vi "test_read-nmea-data2.vi"() -> ()   [LabVIEW 2019] (continued)
,1,04,11,50,132,25,14,87,127,24,28,,,21,33,60,219,29,1*46\n\t\n15:12:35.67\tF9P\t$GBGSV,1,1,03,11,50,132,,14,87,127,33,33,60,219,,3*40\n\t\n15:12:35.69\tF9P\t$GNGLL,3723.54317,N,12656.94702,E,061237.00,A,A*79\n\t\n15:12:35.71\tF9P\t\t\n15:12:35.73\tF9P\t\t\n15:12:35.75\tF9P\t\t\n15:12:35.77\tF9P\t\t\n15:12:35.79\tF9P\t\t\n15:12:35.81\tF9P\t\t\n15:12:35.83\tF9P\t\t\n15:12:35.85\tF9P\t\t\n15:12:35.87\tF9P\t\t\n15:12:35.89\tF9P\t\t\n15:12:35.91\tF9P\t\t\n15:12:35.93\tF9P\t\t\n15:12:35.95\tF9P\t\t\n15:12:35.97\tF9P\t\t\n15:12:35.99\tF9P\t\t\n15:12:36.01\tF9P\t\t\n15:12:36.03\tF9P\t\t\n15:12:36.05\tF9P\t\t\n15:12:36.07\tF9P\t\t\n15:12:36.09\tF9P\t\t\n15:12:36.11\tF9P\t\t\n15:12:36.13\tF9P\t\t\n15:12:36.15\tF9P\t\t\n15:12:36.17\tF9P\t\t\n15:12:36.19\tF9P\t\t\n15:12:36.21\tF9P\t\t\n15:12:36.23\tF9P\t$GNRMC,061238.00,A,3723.54347,N,12656.94820,E,2.767,70.74,250720,,,A,V*33\n\t\n15:12:36.25\tF9P\t$GNVTG,70.74,T,,M,2.767,N,5.124,K,A*11\n\t\n15:12:36.27\tF9P\t$GNGGA,061238.00,3723.54347,N,12656.94820,E,1,12,0.86,47.3,M,18.5,M,,*78\n\t\n15:12:36.29\tF9P\t$GNGSA,A,3,12,06,19,05,17,09,04,02,,,,,1.43,0.86,1.14,1*0C\n\t\n15:12:36.31\tF9P\t$GNGSA,A,3,85,70,71,84,,,,,,,,,1.43,0.86,1.14,2*0E\n\t\n15:12:36.33\tF9P\t$GNGSA,A,3,36,19,11,04,09,12,,,,,,,1.43,0.86,1.14,3*0C\n\t\n15:12:36.35\tF9P\t$GNGSA,A,3,14,11,33,,,,,,,,,,1.43,0.86,1.14,4*0D\n\t\n15:12:36.37\tF9P\t$GPGSV,3,1,09,02,55,319,20,04,18,043,24,05,37,247,38,06,64,049,28,1*60\n\t\n15:12:36.39\tF9P\t$GPGSV,3,2,09,09,45,074,32,12,23,276,30,17,33,154,35,19,52,157,30,1*6B\n\t\n15:12:36.41\tF9P\t$GPGSV,3,3,09,25,12,306,,1*5C\n\t\n15:12:36.43\tF9P\t$GPGSV,3,1,09,02,55,319,,04,18,043,18,05,37,247,21,06,64,049,28,6*62\n\t\n15:12:36.45\tF9P\t$GPGSV,3,2,09,09,45,074,29,12,23,276,16,17,33,154,27,19,52,157,,6*62\n\t\n15:12:36.47\tF9P\t$GPGSV,3,3,09,25,12,306,,6*5B\n\t\n15:12:36.49\tF9P\t$GLGSV,2,1,08,69,12,031,,70,71,039,33,71,52,205,38,72,04,209,23,1*70\n\t\n15:12:36.51\tF9P\t$GLGSV,2,2,08,77,01,326,,84,20,122,10,85,70,067,41,86,37,330,,1*7C\n\t\n15:12:36.53\tF9P\t$GLGSV,2,1,08,69,12,031,,70,71,039,,71,52,205,24,72,04,209,,3*7E\n\t\n15:12:36.55\tF9P\t$GLGSV,2,2,08,77,01,326,,84,20,122,15,85,70,067,21,86,37,330,,3*7D\n\t\n15:12:36.57\tF9P\t$GAGSV,2,1,08,02,08,297,07,04,66,116,32,09,32,193,39,11,72,359,27,7*7C\n\t\n15:12:36.59\tF9P\t$GAGSV,2,2,08,12,40,103,24,19,26,045,17,25,09,249,,36,26,308,21,7*7B\n\t\n15:12:36.61\tF9P\t$GAGSV,2,1,08,02,08,297,,04,66,116,,09,32,193,,11,72,359,,2*70\n\t\n15:12:36.63\tF9P\t$GAGSV,2,2,08,12,40,103,,19,26,045,,25,09,249,,36,26,308,,2*7D\n\t\n15:12:36.65\tF9P\t$GBGSV,1,1,04,11,50,132,26,14,87,127,26,28,,,20,33,60,219,36,1*48\n\t\n15:12:36.67\tF9P\t$GBGSV,1,1,03,11,50,132,,14,87,127,28,33,60,219,,3*4A\n\t\n15:12:36.69\tF9P\t$GNGLL,3723.54347,N,12656.94820,E,061238.00,A,A*7C\n\t\n15:12:36.71\tF9P\t\t\n15:12:36.73\tF9P\t\t\n15:12:36.75\tF9P\t\t\n15:12:36.78\tF9P\t\t\n15:12:36.80\tF9P\t\t\n15:12:36.82\tF9P\t\t\n15:12:36.84\tF9P\t\t\n15:12:36.86\tF9P\t\t\n15:12:36.88\tF9P\t\t\n15:12:36.90\tF9P\t\t\n15:12:36.92\tF9P\t\t\n15:12:36.94\tF9P\t\t\n15:12:36.96\tF9P\t\t\n15:12:36.98\tF9P\t\t\n15:12:37.00\tF9P\t\t\n15:12:37.02\tF9P\t\t\n15:12:37.04\tF9P\t\t\n15:12:37.06\tF9P\t\t\n15:12:37.08\tF9P\t\t\n15:12:37.10\tF9P\t\t\n15:12:37.12\tF9P\t\t\n15:12:37.14\tF9P\t\t\n15:12:37.16\tF9P\t\t\n15:12:37.18\tF9P\t\t\n15:12:37.20\tF9P\t\t\n15:12:37.22\tF9P\t\t\n15:12:37.24\tF9P\t$GNRMC,061239.00,A,3723.54405,N,12656.94928,E,3.255,61.63,250720,,,A,V*39\n\t\n15:12:37.26\tF9P\t$GNVTG,61.63,T,,M,3.255,N,6.028,K,A*1C\n\t\n15:12:37.28\tF9P\t$GNGGA,061239.00,3723.54405,N,12656.94928,E,1,12,0.86,46.9,M,18.5,M,,*7A\n\t\n15:12:37.30\tF9P\t$GNGSA,A,3,12,06,19,05,17,09,04,02,,,,,1.43,0.86,1.14,1*0C\n\t\n15:12:37.32\tF9P\t$GNGSA,A,3,85,70,71,84,,,,,,,,,1.43,0.86,1.14,2*0E\n\t\n15:12:37.34\tF9P\t$GNGSA,A,3,36,19,11,04,09,12,,,,,,,1.43,0.86,1.14,3*0C\n\t\n15:12:37.36\tF9P\t$GNGSA,A,3,14,11,33,,,,,,,,,,1.43,0.86,1.14,4*0D\n\t\n15:12:37.38\tF9P\t$GPGSV,3,1,09,02,55,319,23,04,18,043,24,05,37,247,35,06,64,049,31,1*66\n\t\n15:12:37.40\tF9P\t$GPGSV,3,2,09,09,45,074,30,12,23,276,29,17,33,154,29,19,52,157,34,1*68\n\t\n15:12:37.42\tF9P\t$GPGSV,3,3,09,25,12,306,25,1*5B\n\t\n15:12:37.44\tF9P\t$GPGSV,3,1,09,02,55,319,,04,18,043,19,05,37,247,20,06,64,049,28,6*62\n\t\n15:12:37.46\tF9P\t$GPGSV,3,2,09,09,45,074,32,12,23,276,16,17,33,154,26,19,52,157,,6*69\n\t\n15:12:37.48\tF9P\t$GPGSV,3,3,09,25,12,306,,6*5B\n\t\n15:12:37.50\tF9P\t$GLGSV,2,1,08,69,12,031,,70,71,039,33,71,52,205,43,72,04,209,22,1*7D\n\t\n15:12:37.52\tF9P\t$GLGSV,2,2,08,77,01,326,,84,20,122,14,85,70,067,36,86,37,330,,1*78\n\t\n15:12:37.54\tF9P\t$GLGSV,2,1,08,69,12,031,,70,71,039,,71,52,205,24,72,04,209,,3*7E\n\t\n15:12:37.56\tF9P\t$GLGSV,2,2,08,77,01,326,,84,20,122,16,85,70,067,29,86,37,330,,3*76\n\t\n15:12:37.58\tF9P\t$GAGSV,2,1,08,02,08,297,13,04,66,116,27,09,32,193,33,11,72,359,32,7*73\n\t\n15:12:37.60\tF9P\t$GAGSV,2,2,08,12,40,103,35,19,26,045,17,25,09,249,,36,26,308,24,7*7E\n\t\n15:12:37.62\tF9P\t$GAGSV,2,1,08,02,08,297,,04,66,116,,09,32,193,,11,72,359,,2*70\n\t\n15:12:37.64\tF9P\t$GAGSV,2,2,08,12,40,103,,19,26,045,,25,09,249,,36,26,308,,2*7D\n\t\n15:12:37.66\tF9P\t$GBGSV,1,1,04,11,50,132,27,14,87,127,32,28,,,21,33,60,219,37,1*4C\n\t\n15:12:37.68\tF9P\t$GBGSV,1,1,03,11,50,132,,14,87,127,28,33,60,219,,3*4A\n\t\n15:12:37.70\tF9P\t$GNGLL,3723.54405,N,12656.94928,E,061239.00,A,A*75\n\t\n15:12:37.72\tF9P\t\t\n15:12:37.74\tF9P\t\t\n15:12:37.76\tF9P\t\t\n15:12:37.78\tF9P\t\t\n15:12:37.80\tF9P\t\t\n15:12:37.82\tF9P\t\t\n15:12:37.84\tF9P\t\t\n15:12:37.86\tF9P\t\t\n15:12:37.88\tF9P\t\t\n15:12:37.90\tF9P\t\t\n15:12:37.92\tF9P\t\t\n15:12:37.94\tF9P\t\t\n15:12:37.96\tF9P\t\t\n15:12:37.98\tF9P\t\t\n15:12:38.00\tF9P\t\t\n15:12:38.02\tF9P\t\t\n15:12:38.04\tF9P\t\t\n15:12:38.06\tF9P\t\t\n15:12:38.08\tF9P\t\t\n15:12:38.10\tF9P\t\t\n15:12:38.12\tF9P\t\t\n15:12:38.14\tF9P\t\t\n15:12:38.16\tF9P\t\t\n15:12:38.18\tF9P\t\t\n15:12:38.20\tF9P\t\t\n15:12:38.22\tF9P\t\t\n15:12:38.24\tF9P\t$GNRMC,061240.00,A,3723.54439,N,12656.95015,E,2.349,62.25,250720,,,A,V*32\n\t\n15:12:38.26\tF9P\t$GNVTG,62.25,T,,M,2.349,N,4.351,K,A*1F\n\t\n15:12:38.28\tF9P\t$GNGGA,061240.00,3723.54439,N,12656.95015,E,1,12,0.90,47.7,M,18.5,M,,*75\n\t\n15:12:38.30\tF9P\t$GNGSA,A,3,12,06,19,05,17,09,04,02,,,,,1.51,0.90,1.21,1*0E\n\t\n15:12:38.32\tF9P\t$GNGSA,A,3,85,70,71,84,,,,,,,,,1.51,0.90,1.21,2*0C\n\t\n15:12:38.34\tF9P\t$GNGSA,A,3,36,19,11,04,09,12,,,,,,,1.51,0.90,1.21,3*0E\n\t\n15:12:38.36\tF9P\t$GNGSA,A,3,14,11,33,,,,,,,,,,1.51,0.90,1.21,4*0F\n\t\n15:12:38.38\tF9P\t$GPGSV,3,1,09,02,55,319,25,04,18,043,23,05,37,247,29,06,64,049,32,1*69\n\t\n15:12:38.40\tF9P\t$GPGSV,3,2,09,09,45,074,29,12,23,276,21,17,33,154,36,19,52,157,33,1*61\n\t\n15:12:38.42\tF9P\t$GPGSV,3,3,09,25,12,306,22,1*5C\n\t\n15:12:38.44\tF9P\t$GPGSV,3,1,09,02,55,319,,04,18,043,17,05,37,247,21,06,64,049,28,6*6D\n\t\n15:12:38.46\tF9P\t$GPGSV,3,2,09,09,45,074,27,12,23,276,14,17,33,154,25,19,52,157,,6*6C\n\t\n15:12:38.48\tF9P\t$GPGSV,3,3,09,25,12,306,,6*5B\n\t\n15:12:38.50\tF9P\t$GLGSV,2,1,08,69,12,031,,70,71,039,33,71,52,205,45,72,04,209,20,1*79\n\t\n15:12:38.52\tF9P\t$GLGSV,2,2,08,77,01,326,,84,20,122,10,85,70,067,32,86,37,330,,1*78\n\t\n15:12:38.54\tF9P\t$GLGSV,2,1,08,69,12,031,,70,71,039,,71,52,205,24,72,04,209,,3*7E\n\t\n15:12:38.56\tF9P\t$GLGSV,2,2,08,77,01,326,,84,20,122,17,85,70,067,24,86,37,330,,3*7A\n\t\n15:12:38.58\tF9P\t$GAGSV,2,1,08,02,08,297,12,04,66,116,27,09,32,193,30,11,72,359,31,7*72\n\t\n15:12:38.60\tF9P\t$GAGSV,2,2,08,12,40,103,31,19,26,045,17,25,09,249,,36,26,308,23,7*7D\n\t\n15:12:38.62\tF9P\t$GAGSV,2,1,08,02,08,297,,04,66,116,,09,32,193,,11,72,359,,2*70\n\t\n15:12:38.64\tF9P\t$GAGSV,2,2,08,12,40,103,,19,26,045,,25,09,249,,36,26,308,,2*7D\n\t\n15:12:38.66\tF9P\t$GBGSV,1,1,04,11,50,132,28,14,87,127,28,28,,,23,33,60,219,31,1*4C\n\t\n15:12:38.68\tF9P\t$GBGSV,1,1,03,11,50,132,,14,87,127,26,33,60,219,,3*44\n\t\n15:12:38.70\tF9P\t$GNGLL,3723.54439,N,12656.95015,E,061240.00,A,A*72\n\t\n15:12:38.72\tF9P\t\t\n15:12:38.74\tF9P\t\t\n15:12:38.76\tF9P\t\t\n15:12:38.78\tF9P\t\t\n15:12:38.80\tF9P\t\t\n15:12:38.82\tF9P\t\t\n15:12:38.84\tF9P\t\t\n15:12:38.86\tF9P\t\t\n15:12:38.88\tF9P\t\t\n15:12:38.90\tF9P\t\t\n15:12:38.92\tF9P\t\t\n15:12:38.94\tF9P\t\t\n15:12:38.96\tF9P\t\t\n15:12:38.98\tF9P\t\t\n15:12:39.00\tF9P\t\t\n15:12:39.02\tF9P\t\t\n15:12:39.04\tF9P\t\t\n15:12:39.06\tF9P\t\t\n15:12:39.08\tF9P\t\t\n15:12:39.10\tF9P\t\t\n15:12:39.12\tF9P\t\t\n15:12:39.14\tF9P\t\t\n15:12:39.16\tF9P\t\t\n15:12:39.18\tF9P\t\t\n15:12:39.20\tF9P\t\t\n15:12:39.22\tF9P\t\t\n15:12:39.24\tF9P\t$GNRMC,061241.00,A,3723.54500,N,12656.95069,E,3.058,25.00,250720,,,A,V*35\n\t\n15:12:39.26\tF9P\t$GNVTG,25.00,T,,M,3.058,N,5.663,K,A*1C\n\t\n15:12:39.28\tF9P\t$GNGGA,061241.00,3723.54500,N,12656.95069,E,1,12,0.82,49.2,M,18.5,M,,*7C\n\t\n15:12:39.30\tF9P\t$GNGSA,A,3,12,06,19,05,17,09,04,02,,,,,1.45,0.82,1.20,1*09\n\t\n15:12:39.32\tF9P\t$GNGSA,A,3,85,70,71,84,,,,,,,,,1.45,0.82,1.20,2*0B\n\t\n15:12:39.34\tF9P\t$GNGSA,A,3,36,19,11,04,09,12,,,,,,,1.45,0.82,1.20,3*09\n\t\n15:12:39.36\tF9P\t$GNGSA,A,3,14,11,33,,,,,,,,,,1.45,0.82,1.20,4*08\n\t\n15:12:39.38\tF9P\t$GPGSV,3,1,09,02,55,319,32,04,18,043,23,05,37,247,33,06,64,049,33,1*65\n\t\n15:12:39.40\tF9P\t$GPGSV,3,2,09,09,45,074,30,12,23,276,21,17,33,154,33,19,52,157,26,1*68\n\t\n15:12:39.42\tF9P\t$GPGSV,3,3,09,25,12,306,21,1*5F\n\t\n15:12:39.44\tF9P\t$GPGSV,3,1,09,02,55,319,,04,18,043,16,05,37,247,21,06,64,049,29,6*6D\n\t\n15:12:39.46\tF9P\t$GPGSV,3,2,09,09,45,074,32,12,23,276,12,17,33,154,25,19,52,157,,6*6E\n\t\n15:12:39.48\tF9P\t$GPGSV,3,3,09,25,12,306,,6*5B\n\t\n15:12:39.50\tF9P\t$GLGSV,2,1,08,69,12,031,,70,71,039,33,71,52,205,38,72,04,209,23,1*70\n\t\n15:12:39.52\tF9P\t$GLGSV,2,2,08,77,01,326,,84,20,122,08,85,70,067,38,86,37,330,,1*7B\n\t\n15:12:39.54\tF9P\t$GLGSV,2,1,08,69,12,031,,70,71,039,,71,52,205,22,72,04,209,,3*78\n\t\n15:12:39.56\tF9P\t$GLGSV,2,2,08,77,01,326,,84,20,122,17,85,70,067,23,86,37,330,,3*7D\n\t\n15:12:39.58\tF9P\t$GAGSV,2,1,08,02,08,297,11,04,66,116,26,09,32,193,31,11,72,359,32,7*72\n\t\n15:12:39.60\tF9P\t$GAGSV,2,2,08,12,40,103,31,19,26,045,16,25,09,249,,36,26,308,22,7*7D\n\t\n15:12:39.62\tF9P\t$GAGSV,2,1,08,02,08,297,,04,66,116,,09,32,193,,11,72,359,,2*70\n\t\n15:12:39.64\tF9P\t$GAGSV,2,2,08,12,40,103,,19,26,045,,25,09,249,,36,26,308,,2*7D\n\t\n15:12:39.66\tF9P\t$GBGSV,1,1,04,11,50,132,26,14,87,127,28,28,,,29,33,60,219,33,1*4A\n\t\n15:12:39.68\tF9P\t$GBGSV,1,1,03,11,50,132,,14,87,127,30,33,60,219,,3*43\n\t\n15:12:39.70\tF9P\t$GNGLL,3723.54500,N,12656.95069,E,061241.00,A,A*73\n\t\n15:12:39.72\tF9P\t\t\n15:12:39.74\tF9P\t\t\n15:12:39.76\tF9P\t\t\n15:12:39.78\tF9P\t\t\n15:12:39.80\tF9P\t\t\n15:12:39.82\tF9P\t\t\n15:12:39.84\tF9P\t\t\n15:12:39.86\tF9P\t\t\n15:12:39.88\tF9P\t\t\n15:12:39.90\tF9P\t\t\n15:12:39.92\tF9P\t\t\n15:12:39.94\tF9P\t\t\n15:12:39.96\tF9P\t\t\n15:12:39.98\tF9P\t\t\n15:12:40.00\tF9P\t\t\n15:12:40.02\tF9P\t\t\n15:12:40.04\tF9P\t\t\n15:12:40.06\tF9P\t\t\n15:12:40.08\tF9P\t\t\n15:12:40.10\tF9P\t\t\n15:12:40.12\tF9P\t\t\n15:12:40.14\tF9P\t\t\n15:12:40.16\tF9P\t\t\n15:12:40.18\tF9P\t\t\n15:12:40.20\tF9P\t\t\n15:12:40.22\tF9P\t\t\n15:12:40.24\tF9P\t$GNRMC,061242.00,A,3723.54545,N,12656.95138,E,2.338,43.76,250720,,,A,V*37\n\t\n15:12:40.26\tF9P\t$GNVTG,43.76,T,,M,2.338,N,4.331,K,A*1A\n\t\n15:12:40.28\tF9P\t$GNGGA,061242.00,3723.54545,N,12656.95138,E,1,12,0.82,49.2,M,18.5,M,,*7B\n\t\n15:12:40.30\tF9P\t$GNGSA,A,3,12,06,19,05,17,09,04,02,,,,,1.45,0.82,1.20,1*09\n\t\n15:12:40.32\tF9P\t$GNGSA,A,3,85,70,71,84,,,,,,,,,1.45,0.82,1.20,2*0B\n\t\n15:12:40.34\tF9P\t$GNGSA,A,3,36,19,11,04,09,12,,,,,,,1.45,0.82,1.20,3*09\n\t\n15:12:40.36\tF9P\t$GNGSA,A,3,14,11,33,,,,,,,,,,1.45,0.82,1.20,4*08\n\t\n15:12:40.38\tF9P\t$GPGSV,3,1,09,02,55,319,39,04,18,043,29,05,37,247,36,06,64,049,31,1*63\n\t\n15:12:40.40\tF9P\t$GPGSV,3,2,09,09,45,074,33,12,23,276,23,17,33,154,33,19,52,157,35,1*6B\n\t\n15:12:40.42\tF9P\t$GPGSV,3,3,09,25,12,306,20,1*5E\n\t\n15:12:40.44\tF9P\t$GPGSV,3,1,09,02,55,319,,04,18,043,15,05,37,247,22,06,64,049,28,6*6C\n\t\n15:12:40.46\tF9P\t$GPGSV,3,2,09,09,45,074,28,12,23,276,14,17,33,154,25,19,52,157,,6*63\n\t\n15:12:40.48\tF9P\t$GPGSV,3,3,09,25,12,306,,6*5B\n\t\n15:12:40.50\tF9P\t$GLGSV,2,1,08,69,12,031,23,70,71,039,33,71,52,205,43,72,04,209,23,1*7D\n\t\n15:12:40.52\tF9P\t$GLGSV,2,2,08,77,01,326,,84,20,122,11,85,70,067,33,86,37,330,,1*78\n\t\n15:12:40.54\tF9P\t$GLGSV,2,1,08,69,12,031,,70,71,039,,71,52,205,20,72,04,209,,3*7A\n\t\n15:12:40.56\tF9P\t$GLGSV,2,2,08,77,01,326,,84,20,122,18,85,70,067,29,86,37,330,,3*78\n\t\n15:12:40.58\tF9P\t$GAGSV,2,1,08,02,08,297,14,04,66,116,26,09,32,193,35,11,72,359,35,7*74\n\t\n15:12:40.60\tF9P\t$GAGSV,2,2,08,12,40,103,26,19,26,045,15,25,09,249,,36,26,308,20,7*7A\n\t\n15:12:40.62\tF9P\t$GAGSV,2,1,08,02,08,297,,04,66,116,,09,32,193,,11,72,359,,2*70\n\t\n15:12:40.64\tF9P\t$GAGSV,2,2,08,12,40,103,,19,26,045,,25,09,249,,36,26,308,,2*7D\n\t\n15:12:40.66\tF9P\t$GBGSV,1,1,04,11,50,132,26,14,87,127,29,28,,,38,33,60,219,34,1*4C\n\t\n15:12:40.68\tF9P\t$GBGSV,1,1,03,11,50,132,,14,87,127,29,33,60,219,,3*4B\n\t\n15:12:40.70\tF9P\t$GNGLL,3723.54545,N,12656.95138,E,061242.00,A,A*74\n\t\n15:12:40.72\tF9P\t\t\n15:12:40.74\tF9P\t\t\n15:12:40.76\tF9P\t\t\n15:12:40.78\tF9P\t\t\n15:12:40.80\tF9P\t\t\n15:12:40.82\tF9P\t\t\n15:12:40.84\tF9P\t\t\n15:12:40.86\tF9P\t\t\n15:12:40.88\tF9P\t\t\n15:12:40.90\tF9P\t\t\n15:12:40.92\tF9P\t\t\n15:12:40.94\tF9P\t\t\n15:12:40.96\tF9P\t\t\n15:12:40.98\tF9P\t\t\n15:12:41.00\tF9P\t\t\n15:12:41.02\tF9P\t\t\n15:12:41.04\tF9P\t\t\n15:12:41.06\tF9P\t\t\n15:12:41.08\tF9P\t\t\n15:12:41.10\tF9P\t\t\n15:12:41.12\tF9P\t\t\n15:12:41.14\tF9P\t\t\n15:12:41.16\tF9P\t\t\n15:12:41.18\tF9P\t\t\n15:12:41.20\tF9P\t\t\n15:12:41.22\tF9P\t\t\n15:12:41.24\tF9P\t$GNRMC,061243.00,A,3723.54595,N,12656.95226,E,2.215,50.75,250720,,,A,V*38\n\t\n15:12:41.26\tF9P\t$GNVTG,50.75,T,,M,2.215,N,4.102,K,A*17\n\t\n15:12:41.28\tF9P\t$GNGGA,061243.00,3723.54595,N,12656.95226,E,1,12,0.82,48.7,M,18.5,M,,*7F\n\t\n15:12:41.30\tF9P\t$GNGSA,A,3,12,06,19,05,17,09,04,02,,,,,1.45,0.82,1.20,1*09\n\t\n15:12:41.32\tF9P\t$GNGSA,A,3,85,70,71,84,,,,,,,,,1.45,0.82,1.20,2*0B\n\t\n15:12:41.34\tF9P\t$GNGSA,A,3,36,19,11,04,09,12,,,,,,,1.45,0.82,1.20,3*09\n\t\n15:12:41.36\tF9P\t$GNGSA,A,3,14,11,33,,,,,,,,,,1.45,0.82,1.20,4*08\n\t\n15:12:41.38\tF9P\t$GPGSV,3,1,09,02,55,319,43,04,18,043,27,05,37,247,37,06,64,049,25,1*64\n\t\n15:12:41.40\tF9P\t$GPGSV,3,2,09,09,45,074,35,12,23,276,24,17,33,154,34,19,52,157,33,1*6B\n\t\n15:12:41.42\tF9P\t$GPGSV,3,3,09,25,12,306,20,1*5E\n\t\n15:12:41.44\tF9P\t$GPGSV,3,1,09,02,55,319,,04,18,043,14,05,37,247,22,06,64,049,27,6*62\n\t\n15:12:41.46\tF9P\t$GPGSV,3,2,09,09,45,074,32,12,23,276,12,17,33,154,24,19,52,157,,6*6F\n\t\n15:12:41.48\tF9P\t$GPGSV,3,3,09,25,12,306,,6*5B\n\t\n15:12:41.50\tF9P\t$GLGSV,2,1,08,69,12,031,24,70,71,039,34,71,52,205,43,72,04,209,24,1*7A\n\t\n15:12:41.52\tF9P\t$GLGSV,2,2,08,77,01,326,,84,20,122,13,85,70,067,34,86,37,330,,1*7D\n\t\n15:12:41.54\tF9P\t$GLGSV,2,1,08,69,12,031,,70,71,039,,71,52,205,28,72,04,209,,3*72\n\t\n15:12:41.56\tF9P\t$GLGSV,2,2,08,77,01,326,,84,20,122,19,85,70,067,15,86,37,330,,3*76\n\t\n15:12:41.58\tF9P\t$GAGSV,2,1,08,02,08,297,06,04,66,116,26,09,32,193,39,11,72,359,31,7*7F\n\t\n15:12:41.60\tF9P\t$GAGSV,2,2,08,12,40,103,27,19,26,045,14,25,09,249,,36,26,308,19,7*70\n\t\n15:12:41.62\tF9P\t$GAGSV,2,1,08,02,08,297,,04,66,116,,09,32,193,,11,72,359,,2*70\n\t\n15:12:41.64\tF9P\t$GAGSV,2,2,08,12,40,103,,19,26,045,,25,09,249,,36,26,308,,2*7D\n\t\n15:12:41.66\tF9P\t$GBGSV,1,1,04,11,50,132,27,14,87,127,29,28,,,41,33,60,219,42,1*42\n\t\n15:12:41.68\tF9P\t$GBGSV,1,1,03,11,50,132,,14,87,127,28,33,60,219,,3*4A\n\t\n15:12:41.70\tF9P\t$GNGLL,3723.54595,N,12656.95226,E,061243.00,A,A*74\n\t\n15:12:41.72\tF9P\t\t\n15:12:41.74\tF9P\t\t\n15:12:41.76\tF9P\t\t\n15:12:41.78\tF9P\t\t\n15:12:41.80\tF9P\t\t\n15:12:41.82\tF9P\t\t\n15:12:41.84\tF9P\t\t\n15:12:41.86\tF9P\t\t\n15:12:41.88\tF9P\t\t\n15:12:41.90\tF9P\t\t\n15:12:41.92\tF9P\t\t\n15:12:41.94\tF9P\t\t\n15:12:41.96\tF9P\t\t\n15:12:41.98\tF9P\t\t\n15:12:42.00\tF9P\t\t\n15:12:42.02\tF9P\t\t\n15:12:42.04\tF9P\t\t\n15:12:42.06\tF9P\t\t\n15:12:42.08\tF9P\t\t\n15:12:42.10\tF9P\t\t\n15:12:42.12\tF9P\t\t\n15:12:42.14\tF9P\t\t\n15:12:42.16\tF9P\t\t\n15:12:42.18\tF9P\t\t\n15:12:42.20\tF9P\t\t\n15:12:42.22\tF9P\t\t\n15:12:42.24\tF9P\t$GNRMC,061244.00,A,3723.54642,N,12656.95297,E,2.119,51.11,250720,,,A,V*30\n\t\n15:12:42.26\tF9P\t$GNVTG,51.11,T,,M,2.119,N,3.925,K,A*11\n\t\n15:12:42.28\tF9P\t$GNGGA,061244.00,3723.54642,N,12656.95297,E,1,12,0.82,48.7,M,18.5,M,,*7B\n\t\n15:12:42.30\tF9P\t$GNGSA,A,3,12,06,19,05,17,09,04,02,,,,,1.45,0.82,1.20,1*09\n\t\n15:12:42.32\tF9P\t$GNGSA,A,3,85,70,71,84,,,,,,,,,1.45,0.82,1.20,2*0B\n\t\n15:12:42.34\tF9P\t$GNGSA,A,3,36,19,11,04,09,12,,,,,,,1.45,0.82,1.20,3*09\n\t\n15:12:42.36\tF9P\t$GNGSA,A,3,14,11,33,,,,,,,,,,1.45,0.82,1.20,4*08\n\t\n15:12:42.38\tF9P\t$GPGSV,3,1,09,02,55,319,37,04,18,043,26,05,37,247,32,06,64,049,33,1*64\n\t\n15:12:42.40\tF9P\t$GPGSV,3,2,09,09,45,074,29,12,23,276,23,17,33,154,34,19,52,157,28,1*6B\n\t\n15:12:42.42\tF9P\t$GPGSV,3,3,09,25,12,306,21,1*5F\n\t\n15:12:42.44\tF9P\t$GPGSV,3,1,09,02,55,319,,04,18,043,15,05,37,247,22,06,64,049,26,6*62\n\t\n15:12:42.46\tF9P\t$GPGSV,3,2,09,09,45,074,27,12,23,276,,17,33,154,24,19,52,157,,6*68\n\t\n15:12:42.48\tF9P\t$GPGSV,3,3,09,25,12,306,,6*5B\n\t\n15:12:42.50\tF9P\t$GLGSV,2,1,08,69,12,031,24,70,71,039,33,71,52,205,47,72,04,209,22,1*7F\n\t\n15:12:42.52\tF9P\t$GLGSV,2,2,08,77,01,326,,84,20,122,11,85,70,067,36,86,37,330,,1*7D\n\t\n15:12:42.54\tF9P\t$GLGSV,2,1,08,69,12,031,,70,71,039,,71,52,205,27,72,04,209,,3*7D\n\t\n15:12:42.56\tF9P\t$GLGSV,2,2,08,77,01,326,,84,20,122,,85,70,067,24,86,37,330,,3*7C\n\t\n15:12:42.58\tF9P\t$GAGSV,2,1,08,02,08,297,14,04,66,116,26,09,32,193,39,11,72,359,37,7*7A\n\t\n15:12:42.60\tF9P\t$GAGSV,2,2,08,12,40,103,26,19,26,045,14,25,09,249,,36,26,308,17,7*7F\n\t\n15:12:42.62\tF9P\t$GAGSV,2,1,08,02,08,297,,04,66,116,,09,32,193,34,11,72,359,,2*77\n\t\n15:12:42.64\tF9P\t$GAGSV,2,2,08,12,40,103,,19,26,045,,25,09,249,,36,26,308,,2*7D\n\t\n15:12:42.66\tF9P\t$GBGSV,1,1,04,11,50,132,26,14,87,127,30,28,,,47,33,60,219,39,1*41\n\t\n15:12:42.68\tF9P\t$GBGSV,1,1,03,11,50,132,,14,87,127,32,33,60,219,,3*41\n\t\n15:12:42.70\tF9P\t$GNGLL,3723.54642,N,12656.95297,E,061244.00,A,A*70\n\t\n15:12:42.72\tF9P\t\t\n15:12:42.74\tF9P\t\t\n15:12:42.76\tF9P\t\t\n15:12:42.78\tF9P\t\t\n15:12:42.80\tF9P\t\t\n15:12:42.82\tF9P\t\t\n15:12:42.84\tF9P\t\t\n15:12:42.86\tF9P\t\t\n15:12:42.88\tF9P\t\t\n15:12:42.90\tF9P\t\t\n15:12:42.92\tF9P\t\t\n15:12:42.94\tF9P\t\t\n15:12:42.96\tF9P\t\t\n15:12:42.98\tF9P\t\t\n15:12:43.00\tF9P\t\t\n15:12:43.02\tF9P\t\t\n15:12:43.04\tF9P\t\t\n15:12:43.06\tF9P\t\t\n15:12:43.08\tF9P\t\t\n15:12:43.10\tF9P\t\t\n15:12:43.12\tF9P\t\t\n15:12:43.14\tF9P\t\t\n15:12:43.16\tF9P\t\t\n15:12:43.18\tF9P\t\t\n15:12:43.20\tF9P\t\t\n15:12:43.22\tF9P\t\t\n15:12:43.24\tF9P\t$GNRMC,061245.00,A,3723.54718,N,12656.95403,E,2.939,50.30,250720,,,A,V*3C\n\t\n15:12:43.26\tF9P\t$GNVTG,50.30,T,,M,2.939,N,5.444,K,A*15\n\t\n15:12:43.28\tF9P\t$GNGGA,061245.00,3723.54718,N,12656.95403,E,1,12,0.95,47.2,M,18.5,M,,*73\n\t\n15:12:43.30\tF9P\t$GNGSA,A,3,12,06,19,05,17,09,04,02,,,,,1.88,0.95,1.62,1*08\n\t\n15:12:43.32\tF9P\t$GNGSA,A,3,85,70,71,84,,,,,,,,,1.88,0.95,1.62,2*0A\n\t\n15:12:43.34\tF9P\t$GNGSA,A,3,36,19,11,04,09,12,,,,,,,1.88,0.95,1.62,3*08\n\t\n15:12:43.36\tF9P\t$GNGSA,A,3,14,11,33,,,,,,,,,,1.88,0.95,1.62,4*09\n\t\n15:12:43.38\tF9P\t$GPGSV,3,1,09,02,55,319,39,04,18,043,,05,37,247,34,06,64,049,27,1*6D\n\t\n15:12:43.40\tF9P\t$GPGSV,3,2,09,09,45,074,36,12,23,276,23,17,33,154,34,19,52,157,28,1*65\n\t\n15:12:43.42\tF9P\t$GPGSV,3,3,09,25,12,306,23,1*5D\n\t\n15:12:43.44\tF9P\t$GPGSV,3,1,09,02,55,319,,04,18,043,16,05,37,247,25,06,64,049,26,6*66\n\t\n15:12:43.46\tF9P\t$GPGSV,3,2,09,09,45,074,36,12,23,276,,17,33,154,25,19,52,157,,6*69\n\t\n15:12:43.48\tF9P\t$GPGSV,3,3,09,25,12,306,,6*5B\n\t\n15:12:43.50\tF9P\t$GLGSV,2,1,08,69,12,031,23,70,71,039,27,71,52,205,46,72,04,209,22,1*7C\n\t\n15:12:43.52\tF9P\t$GLGSV,2,2,08,77,01,326,,84,20,122,09,85,70,067,38,86,37,330,,1*7A
